vi "Check Config File Multilink.vi"(8 "error in (no error)":errorcluster, 9 "Save As?":bool, 10 "Index":i32, 11 "cDAQ Configs":T2[](array[typedef])) -> (0 "error out":errorcluster, 1 "Which Button?":T1(ring), 3 "CfgFile Path":path, 5 "Referencing Chassis":string[](array[string]))   [LabVIEW 2012, in "Configuration Grandmaster.lvlib" / "Cfg Grandmaster.lvclass"]
uses:
  Cfg Grandmaster.lvclass
  Custom Ctrls/Master Cfg/ge_Cfg wChassis.ctl
  Class Chassis Cfg/ChassisCfg.lvclass
  Class Chassis BOM/Chassis BOM.lvclass
  Data Acquisition/Class Chassis Tasks/Chassis Tasks.lvclass
  Class Chassis BOM/Chassis BOM.lvclass/Chassis BOM.ctl
  Class Chassis BOM/Read Chassis Alias.vi
  Class Chassis BOM/Read CfgFile.vi
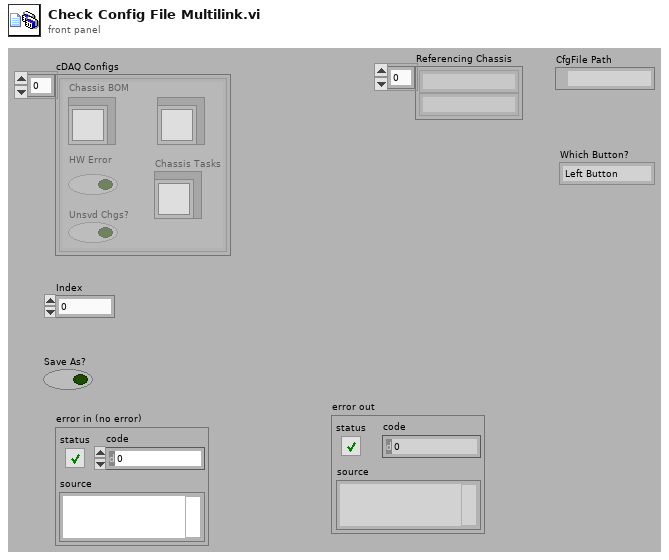
[diagram p1: front panel]
types:
  T1 = enum16{"Left Button", "Center Button", "Right Button", "Window Close"}
  T2 = typedef "ge_Cfg wChassis.ctl" = cluster{"Chassis BOM":refnum<class "Chassis BOM.lvclass">, "Chassis Cfg":refnum<class "ChassisCfg.lvclass">, "Chassis Tasks":refnum<class "Chassis Tasks.lvclass">, "HW Error":bool, "Unsvd Chgs?":bool}
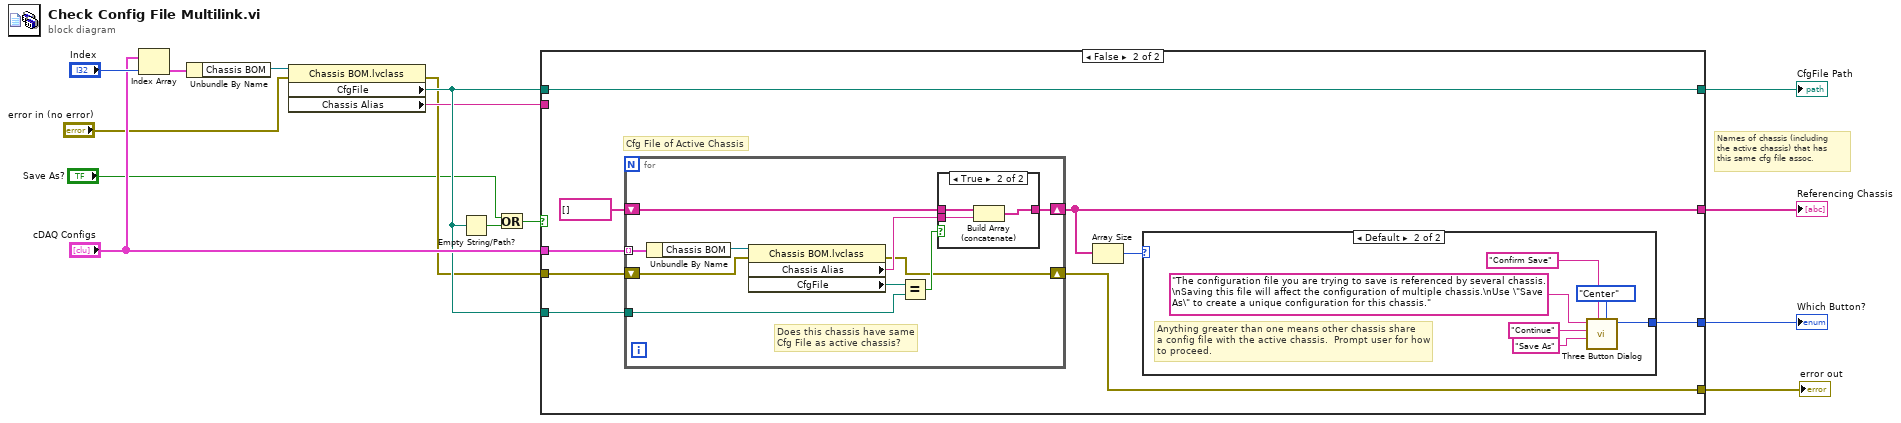
[diagram p0: block diagram]
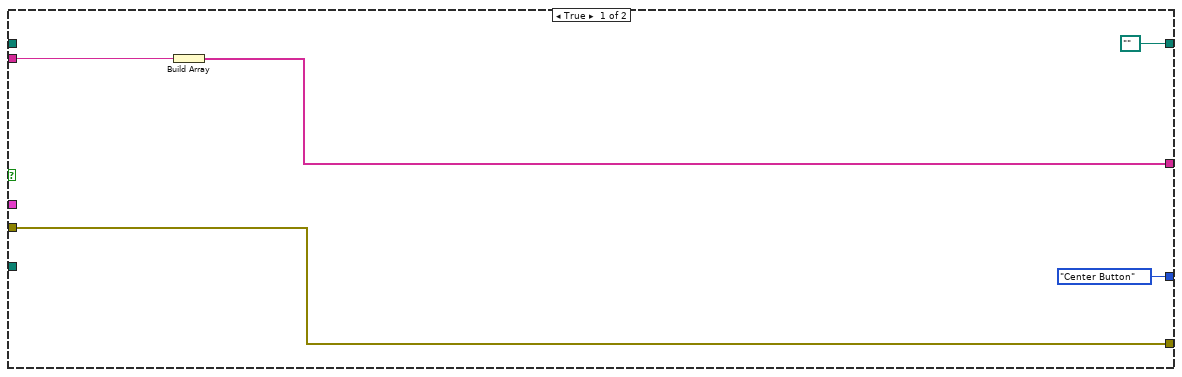
[diagram p2: hidden frame]
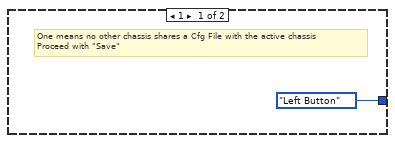
[diagram p3: hidden frame]
diagram:
  # "Names of chassis (including\nthe active chassis) that has\nthis same cfg file assoc."
  n1 = Index Array(array="cDAQ Configs", index="Index") -> (element=w6:T2)
  n2 = Unbundle By Name(w6) -> ("Chassis BOM"=w8:refnum<class "Chassis BOM.lvclass">)
  n3 = property class="Chassis BOM.lvclass"(reference=w8, error in="error in (no error)") -> (error out=w3:errorcluster, "CfgFile"=w7:path, "Chassis Alias"=w5:string)  [unwired: 1 out]
  n4 = Empty String/Path?(string/path=w7) -> (empty?=w9:bool)
  n5 = Or(x="Save As?", y=w9) -> (x .or. y?=w10:bool)
  n6 = case shown="False" w10 {
    tunnel: "cDAQ Configs" -> [_ w29]
    tunnel: [w19 w26] -> w13
    tunnel: w7 -> [_ w27]
    tunnel: w5 -> [w20 _]
    tunnel: [T1."Center Button" ("Which Button?") w24] -> w11
    tunnel: w7 -> [_ w23]
    tunnel: [path "" ("CfgFile") w23] -> w12
    tunnel: w3 -> [w16 w22]
    tunnel: [w16 w21] -> w2
    frame True {
      n7 = Build Array(w20) -> (w19:string[])
    }
    frame False {
      # "Cfg File of Active Chassis"
      n8 = for {
        tunnel: w29 -> [w39] mode=indexing
        tunnel: w27 -> [w46]
        shift-right: [w44] -> w26
        shift-left: string[] [] -> [w45]
        shift-right: [w37] -> w21
        shift-left: w22 -> [w38]
        # "Does this chassis have same \nCfg File as active chassis?"
        n9 = Unbundle By Name(w39) -> ("Chassis BOM"=w42:refnum<class "Chassis BOM.lvclass">)
        n10 = property class="Chassis BOM.lvclass"(reference=w42, error in=w38) -> (error out=w37:errorcluster, "Chassis Alias"=w41:string, "CfgFile"=w40:path)  [unwired: 1 out]
        n11 = Equal?(x=w40, y=w46) -> (x = y?=w43:bool)
        n12 = case shown="True" w43 {
          tunnel: w45 -> [w47 w50]
          tunnel: [w47 w49] -> w44
          tunnel: w41 -> [_ w48]
          frame False {
          }
          frame True {
            n13 = Build Array (concatenate)(w50, w48) -> (w49:string[])
          }
        }
      }
      n14 = Array Size(array=w26) -> (size(s)=w25:i32)
      n15 = case shown="Default" w25 {
        tunnel: [T1."Left Button" ("Which Button?") w32] -> w24
        frame 1 {
          # "One means no other chassis shares a Cfg File with the active chassis\nProceed with \"Save\""
        }
        frame Default {
          # "Anything greater than one means other chassis share\na config file with the active chassis.  Prompt user for how\nto proceed."
          n16 = call <vilib>:"Three Button Dialog.vi"("Justify Message (Left)"=enum16{"Left", "Center", "Right"}."Center", "Window Title (\"\")"="Confirm Save" ("Window Title (\"\")"), "Center Button Text (\"No\")"="Save As" ("Center Button Text (\"No\")"), "Left Button Text (\"Yes\")"="Continue" ("Left Button Text (\"Yes\")"), "message"="The configuration file you are trying to save is referenced by several chassis.\nSaving this file will affect the configuration of multiple chassis.\nUse \"Save As\" to create a unique configuration for this chassis." ("Window Title (\"\")")) -> ("Which Button?"=w32:T1)  [unwired: 6 in]
        }
      }
    }
  }
  "CfgFile Path" <- w12
  "Which Button?" <- w11
  "Referencing Chassis" <- w13
  "error out" <- w2
